vi "IMAQ FPGA Camera Link 2 Tap 8-Bit 2 X-Zones.vi"(6 "Ready for Output":bool=TRUE, 7 "Camera Link Enables":T2, 8 "Cancel Acquisition":bool, 9 "Acquire":bool=TRUE, 10 "Camera Link Data":cluster{"Port A":u8, "Port B":u8}, 11 "Acquisition Settings":T3) -> (0 "Output Valid":bool, 2 "Acquisition Status":T1, 3 "Vision Pixel Bus Out":T4={"Pixel Data"=[0, 0, 0, 0, 0, 0, 0, 0], "DV"=[FALSE, FALSE, FALSE, FALSE, FALSE, FALSE, FALSE, FALSE], "EOL"=FALSE, "EOI"=FALSE, "Data Type"=enum."U8 x 8"}, 5 "Acquisition Overflow":bool)   [LabVIEW 2020]
doc: "Acquires images from a 2 tap Left/Right (2X-1Y) Camera Link Camera. Ensure that this VI is called from a Single Cycle Timed Loop that is running faster than the pixel clock of the camera.\n\nThe <B>Vision Pixel Bus Out</B> can be connected to Vision FPGA algorithms for processing."
uses:
  <vilib>/visionFPGA/Controls/IMAQ FPGA Pixel Bus u8x8.ctl
  <vilib>/visionFPGA/Basics/Camera Link Acquisition/CL Data to Pixels/IMAQ FPGA Camera Link Data to Pixels 2 Tap 8-Bit.vi
  <vilib>/visionFPGA/Basics/Camera Link Acquisition/Line Builder/IMAQ FPGA Camera Link Line Builder (2 Tap U8 2X-1Y).vi
  <vilib>/visionFPGA/Basics/Camera Link Acquisition/Pixel Bus to Vision Pixel Bus/IMAQ FPGA Camera Link Pixel Bus to Vision Pixel Bus U8x8.vi
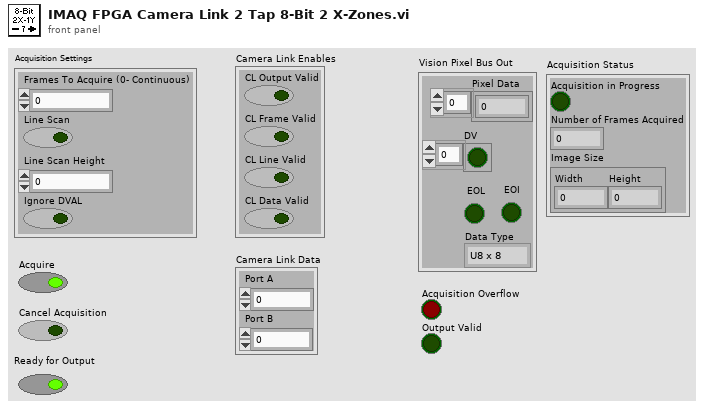
[diagram p1: front panel]
types:
  T1 = cluster{"Acquisition in Progress":bool, "Number of Frames Acquired":u32, "Image Size":cluster{"Width":u32, "Height":u32}}
  T2 = cluster{"CL Output Valid":bool, "CL Frame Valid":bool, "CL Line Valid":bool, "CL Data Valid":bool}
  T3 = cluster{"Frames To Acquire (0- Continuous)":u32, "Line Scan":bool, "Line Scan Height":u32, "Ignore DVAL":bool}
  T4 = typedef "IMAQ FPGA Pixel Bus u8x8.ctl" = cluster{"Pixel Data":u8[], "DV":bool[], "EOL":bool, "EOI":bool, "Data Type":enum16{"U8 x 8"}}
  T5 = cluster{"Acquisition in Progress":bool, "Num Frames Acquired":u32, "Height":u32, "Number of Cycles per Line":u32}
  T6 = cluster{"Acquisition in Progress":bool, "Num Frames Acquired":u32, cluster{u32, "Height":u32}}
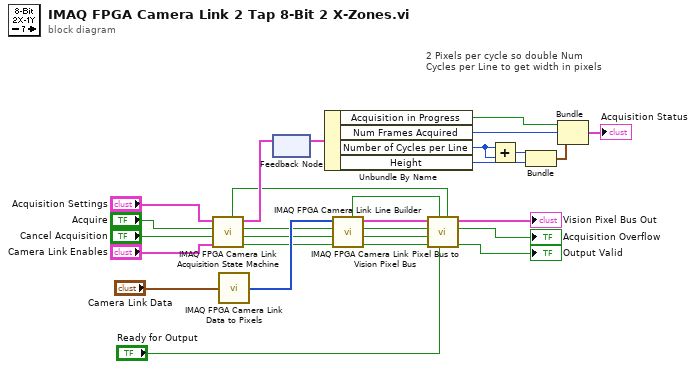
[diagram p0: block diagram]
diagram:
  # "2 Pixels per cycle so double Num Cycles per Line to get width in pixels"
  n1 = call <vilib>:"IMAQ FPGA Camera Link Acquisition State Machine.vi"("Enables"="Camera Link Enables", "Cancel Acq"="Cancel Acquisition", "Acquire"="Acquire", "Acquisition Settings"="Acquisition Settings") -> ("Output Valid"=w7:bool, "Frame Valid"=w8:bool, "Line Valid"=w9:bool, "Acquisition Status"=w25:T5, "Reset"=w18:bool)  [unwired: 3 in]
  n2 = call-poly <vilib>:"IMAQ FPGA Camera Link Data to Pixels.vi"("Camera Link Data"="Camera Link Data") -> ("Pixels"=w10:u8[])
  n3 = feedback #1() -> (w5:T5)  [unwired: 1 in]
  n4 = feedback-in #1(w25) -> ()
  n5 = Unbundle By Name(w5) -> ("Acquisition in Progress"=w4:bool, "Num Frames Acquired"=w3:u32, "Number of Cycles per Line"=w28:u32, "Height"=w27:u32)
  n6 = call-poly <vilib>:"IMAQ FPGA Camera Link Line Builder.vi"("Input Valid In"=w7, "Frame Valid In"=w8, "Line Valid In"=w9, "Pixel Data In"=w10) -> ("Output Valid"=w11:bool, "Frame Valid Out"=w12:bool, "Line Valid Out"=w13:bool, "Pixel Bus x8 Out"=w14:cluster{"Pixels":u8[], "DV":bool[]}, "Overflow"=w22:bool)  [unwired: 3 in]
  n7 = call-poly <vilib>:"IMAQ FPGA Camera Link Pixel Bus to Vision Pixel Bus.vi"("Reset Overflow"=w18, "Ready for Output"="Ready for Output", "Overflow In"=w22, "Input Valid"=w11, "Frame Valid In"=w12, "Line Valid In"=w13, "Pixel Bus x8 In"=w14) -> ("Output Valid"=→"Output Valid":bool, "Acquisition Overflow"=→"Acquisition Overflow":bool, "Vision Pixel Bus Out"=→"Vision Pixel Bus Out":T4)  [unwired: 2 in]
  n8 = Add(x=w28, y=w28) -> (x+y=w26:u32)
  n9 = Bundle(w26, "Height"=w27) -> (w2:cluster{u32, "Height":u32})  [unwired: 1 in]
  n10 = Bundle("Acquisition in Progress"=w4, "Num Frames Acquired"=w3, w2) -> (→"Acquisition Status":T6)  [unwired: 1 in]
